vi "POV Direction.vi"(11 "Value":i32) -> (3 "POV Direction":T1)   [LabVIEW 2020, in "Joystick.lvlib"]
uses:
  Joystick.lvlib
  POV Direction.ctl
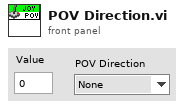
[diagram p1: front panel]
types:
  T1 = typedef "Joystick.lvlib/POV Direction.ctl" = enum16{"None", "Up", "Up Right", "Right", "Down Right", "Down", "Down Left", "Left", "Up Left"}
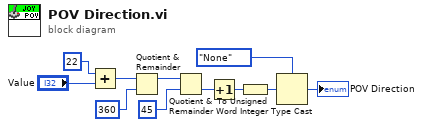
[diagram p0: block diagram]
diagram:
  n1 = Add(x=22, y="Value") -> (x+y=w3:i32)
  n2 = Quotient & Remainder(x=w3, y=360) -> (x-y*floor(x/y)=w2:i32)  [unwired: 1 out]
  n3 = Quotient & Remainder(x=w2, y=45) -> (floor(x/y)=w9:i32)  [unwired: 1 out]
  n4 = Increment(x=w9) -> (x+1=w8:i32)
  n5 = To Unsigned Word Integer(number=w8) -> (unsigned 16bit integer=w5:u16)
  n6 = Type Cast(type=POV_Direction."None" ("POV Direction"), x=w5) -> (*(type *) &x=→"POV Direction":T1)
